vi "Read Encryption.vi"(8 "error in (no error)":errorcluster, 11 "Log Sinks in":refnum<class "Log Sinks.lvclass">) -> (0 "error out":errorcluster, 2 "Encryption":refnum<class "Encryption.lvclass">, 3 "Log Sinks out":refnum<class "Log Sinks.lvclass">)   [LabVIEW 2019, in "TSC Event Logger.lvlib" / "Log Sinks.lvclass"]
doc: "Data member access method to read the encryption type\n\n<b>Code Developed By:</b>\nTechnology Service Corporation\nBloomington, IN 47403\nwww.tsc.com/atcs\n\nDeveloper:\nDaniel Coons"
uses:
  Log Sinks.lvclass
  Encryption/Encryption.lvclass
  Log Sinks.lvclass/Log Sinks.ctl
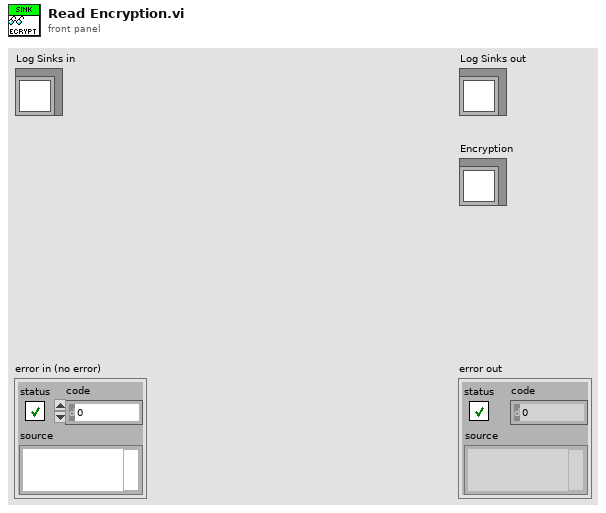
[diagram p1: front panel]
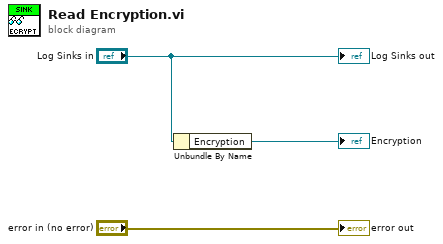
[diagram p0: block diagram]
diagram:
  n1 = Unbundle By Name("Log Sinks in") -> ("Encryption"=→"Encryption":refnum<class "Encryption.lvclass">)
  "error out" <- "error in (no error)"
  "Log Sinks out" <- "Log Sinks in"
